vi "GetCoord.vi"(4 "4":bool, 5 "2":bool, 6 "3":bool, 7 "1":bool, 8 "4":i32, 9 "3":i32, 10 "2":i32, 11 "1":i32) -> (0 "Problem":bool, 1 "INDEX":i32, 2 "OUT":i32)   [LabVIEW 2011]
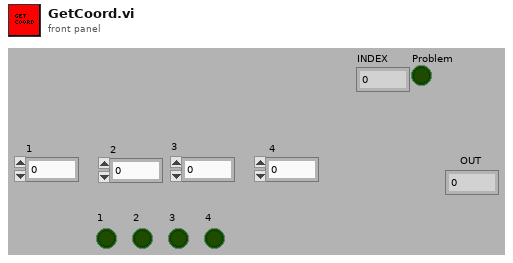
[diagram p1: front panel]
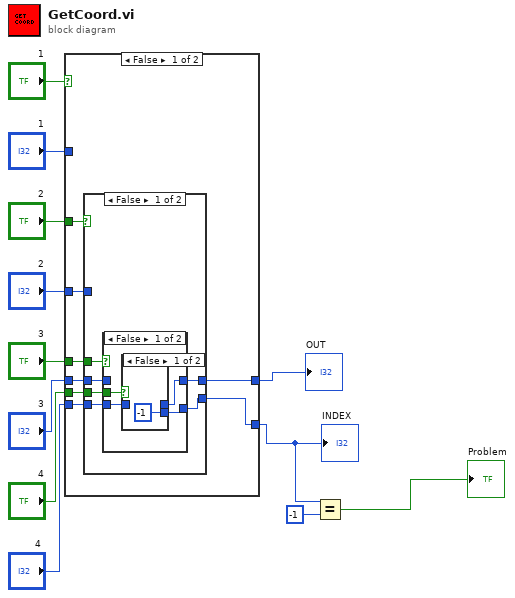
[diagram p0: block diagram]
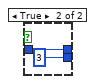
[diagram p2: hidden frame]
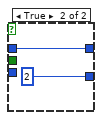
[diagram p3: hidden frame]
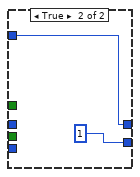
[diagram p4: hidden frame]
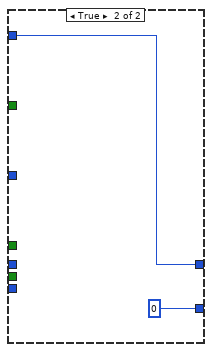
[diagram p5: hidden frame]
diagram:
  n1 = case shown="False" "1" {
    tunnel: "1" -> [_ w39]
    tunnel: [w18 w39] -> w10
    tunnel: "2" -> [w20 _]
    tunnel: "2" -> [w19 _]
    tunnel: "3" -> [w17 _]
    tunnel: "3" -> [w16 _]
    tunnel: "4" -> [w15 _]
    tunnel: "4" -> [w14 _]
    tunnel: [w13 0 ("1")] -> w3
    frame False {
      n2 = case shown="False" w20 {
        tunnel: w19 -> [_ w37]
        tunnel: [w25 w37] -> w18
        tunnel: w17 -> [w26 _]
        tunnel: w16 -> [w24 _]
        tunnel: w15 -> [w23 _]
        tunnel: w14 -> [w22 _]
        tunnel: [w21 1 ("1")] -> w13
        frame False {
          n3 = case shown="False" w26 {
            tunnel: [w29 w35] -> w25
            tunnel: w24 -> [_ w35]
            tunnel: w23 -> [w30 _]
            tunnel: w22 -> [w28 _]
            tunnel: [w27 2 ("1")] -> w21
            frame False {
              n4 = case shown="False" w30 {
                tunnel: [_ w33] -> w29
                tunnel: w28 -> [_ w33]
                tunnel: [-1 ("1") 3 ("1")] -> w27
                frame False {
                }
                frame True {
                }
              }
            }
            frame True {
            }
          }
        }
        frame True {
        }
      }
    }
    frame True {
    }
  }
  "OUT" <- w10
  "INDEX" <- w3
  n5 = Equal?(x=w3, y=-1) -> (x = y?=→"Problem":bool)
